vi "Operator Input.vi"(8 "error in (no error)":errorcluster, 11 "Message":string) -> (0 "error out":errorcluster, 2 "Stop button hit":bool, 3 "Response":string)   [LabVIEW 2013]
panel:
  in  "stop":bool
  in  "Response1":string
  # "Operator Message"
  # "Scan or Enter Response"
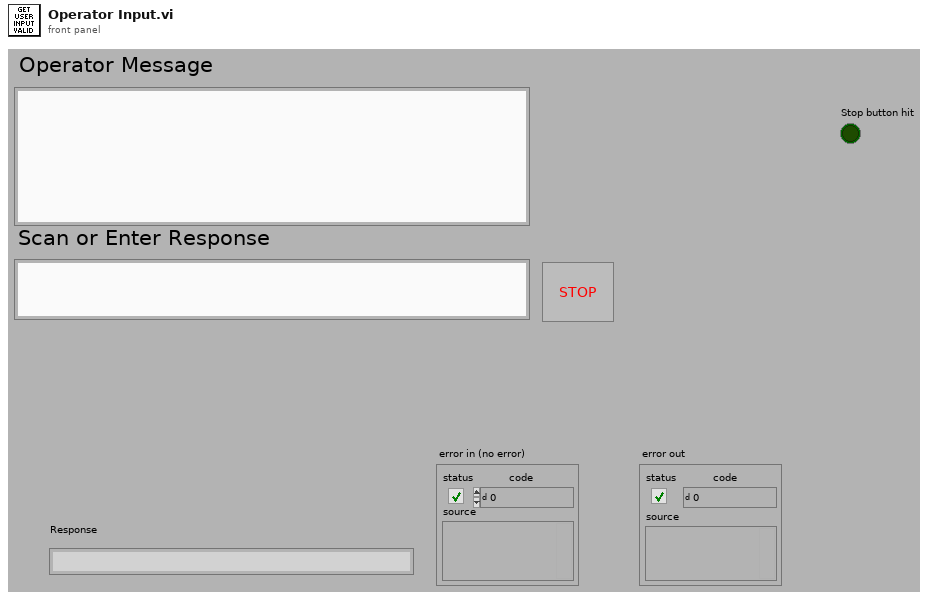
[diagram p1: front panel]
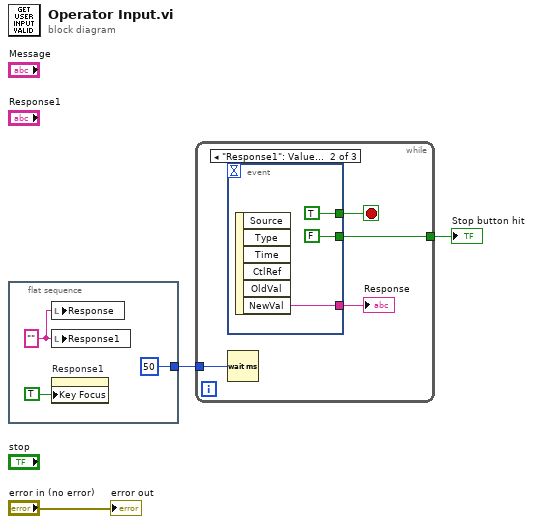
[diagram p0: block diagram]
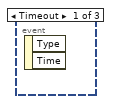
[diagram p2: hidden frame]
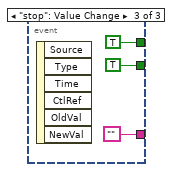
[diagram p3: hidden frame]
diagram:
  n1 = flat-sequence {
    tunnel: [u32 50 ("milliseconds to wait")] -> w3
    frame #0 {
      w4 = "" ("Response1")
      n2 = local write "Response"(w4) -> ()
      n3 = local write "Response1"(w4) -> ()
      n4 = property on="Response1" class="Str"("Key Focus"=TRUE) -> ()  [unwired: 2 in, 2 out]
    }
  }
  n5 = while {
    tunnel: w3 -> [w10]
    tunnel: [w7] -> w1
    stop <- w9 stop-if-true
    n6 = event shown="[1] \"Response1\": Value Change" {
      selector: _ -> [_ _ _]
      dyn-events: _ -> [_ _ _]
      timeout: _ -> [_ _ _]
      tunnel: [_ TRUE TRUE] -> w9
      tunnel: [_ w12 ""] -> w8
      tunnel: [_ FALSE TRUE] -> w7
      event Timeout {
        n7 = event-data() -> ()  [unwired: 1 in, 2 out]
      }
      event "Response1": Value Change {
        n8 = event-data() -> ("NewVal"=w12:string)  [unwired: 1 in, 5 out]
      }
      event "stop": Value Change {
        n9 = event-data() -> ()  [unwired: 1 in, 6 out]
      }
    }
    "Response" <- w8
    n10 = Wait (ms)(milliseconds to wait=w10) -> ()  [unwired: 1 out]
  }
  "Stop button hit" <- w1
  "error out" <- "error in (no error)"
